vi "FlatToRichniswitch_grpc_InitWithOptionsRequest.vi"(5 "OutputClusterType":T1, 11 "InputCluster":T3) -> (3 "OutputCluster":T1)   [LabVIEW 2021, in "NI Switch_client.lvlib"]
uses:
  NI Switch_client.lvlib
  niswitch_grpc_InitWithOptionsRequest_Flat.ctl
  nidevice_grpc_SessionInitializationBehavior.ctl
  niswitch_grpc_InitWithOptionsRequest.ctl
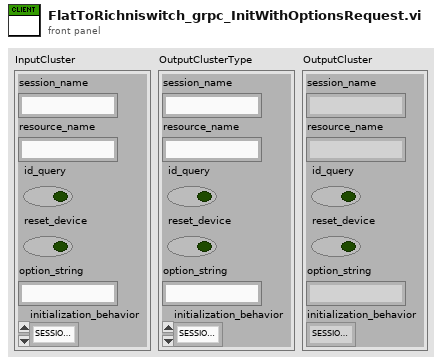
[diagram p1: front panel]
types:
  T1 = typedef "NI Switch_client.lvlib/niswitch_grpc_InitWithOptionsRequest.ctl" = cluster{"session_name":string, "resource_name":string, "id_query":bool, "reset_device":bool, "option_string":string, "initialization_behavior":T2}
  T2 = typedef "NI Switch_client.lvlib/nidevice_grpc_SessionInitializationBehavior.ctl" = enum32{"SESSION_INITIALIZATION_BEHAVIOR_UNSPECIFIED", "SESSION_INITIALIZATION_BEHAVIOR_INITIALIZE_NEW", "SESSION_INITIALIZATION_BEHAVIOR_ATTACH_TO_EXISTING"}
  T3 = typedef "NI Switch_client.lvlib/niswitch_grpc_InitWithOptionsRequest_Flat.ctl" = cluster{"session_name":string, "resource_name":string, "id_query":bool, "reset_device":bool, "option_string":string, "initialization_behavior":T2}
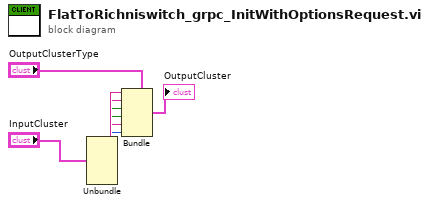
[diagram p0: block diagram]
diagram:
  n1 = Unbundle "Unbundle"("InputCluster") -> ("session_name"=w6:string, "resource_name"=w5:string, "id_query"=w4:bool, "reset_device"=w3:bool, "option_string"=w2:string, "initialization_behavior"=w1:T2)
  n2 = Bundle "Bundle"(cluster="OutputClusterType", "session_name"=w6, "resource_name"=w5, "id_query"=w4, "reset_device"=w3, "option_string"=w2, "initialization_behavior"=w1) -> (→"OutputCluster":T1)
